vi "desktopMain.vi"() -> ()   [LabVIEW 2018]
panel:
  out "웨이브폼 차트":dbl(graph)
  in  "정지 버튼":bool
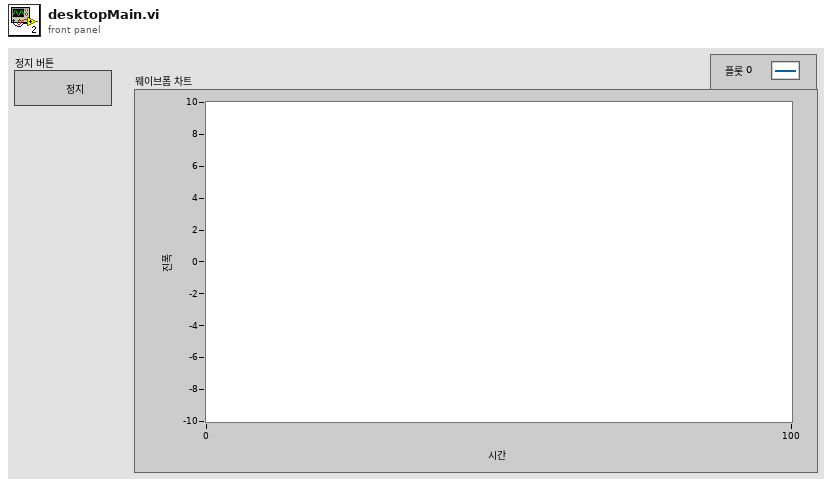
[diagram p1: front panel]
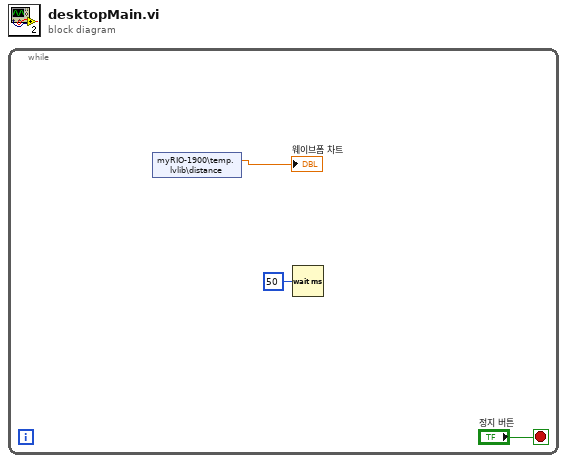
[diagram p0: block diagram]
diagram:
  n1 = while {
    stop <- "정지 버튼" stop-if-true
    n2 = shared-variable "myRIO-1900\\temp.lvlib\\distance"() -> (→"웨이브폼 차트":dbl)  [unwired: 1 in, 1 out]
    n3 = Wait (ms)(milliseconds to wait=u32 50 ("대기 시간 (ms)")) -> ()  [unwired: 1 out]
  }
